vi "Draw_rounded_corners.vi"(7 "Corner scale  factor":dbl=0.1655 format="%#_13g", 8 "error in (no error)":errorcluster, 9 "Inner box coords":T1, 10 "Whole cage size, pix":cluster{"W":dbl, "H":dbl}, 11 "Refnum in":T2) -> (0 "error out":errorcluster, 3 "Refnum out":T2)   [LabVIEW 2018, in "Cage Diagram.lvlib"]
uses:
  Cage Diagram.lvlib
  <vilib>/vision/Image Controls.llb/IMAQ Image.ctl
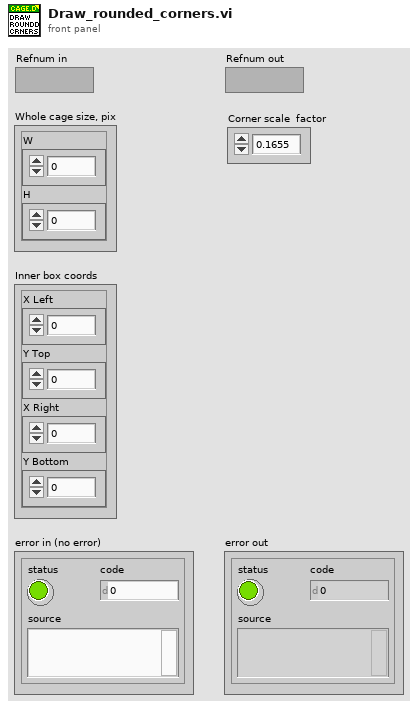
[diagram p1: front panel]
types:
  T1 = cluster{"X Left":dbl, "Y Top":dbl, "X Right":dbl, "Y Bottom":dbl}
  T2 = typedef "IMAQ Image.ctl" = refnum<image>
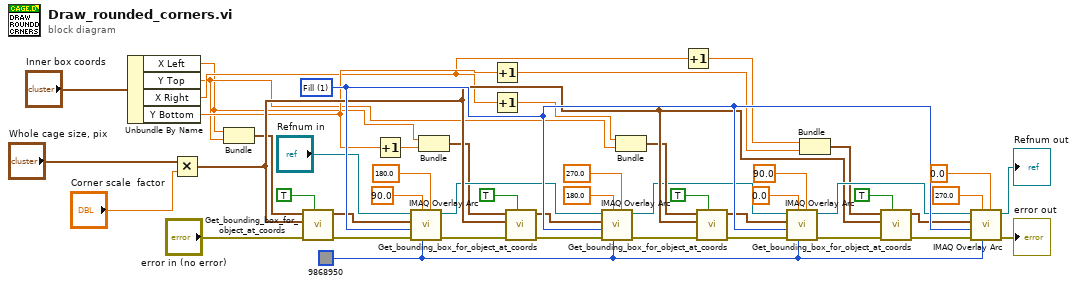
[diagram p0: block diagram]
diagram:
  w48 = u32 9868950 ("Color")
  w47 = u32 1 items=["Frame", "Fill"] ("Drawing Mode (Frame)")
  n1 = Unbundle By Name("Inner box coords") -> ("X Left"=w22:dbl, "Y Top"=w33:dbl, "X Right"=w41:dbl, "Y Bottom"=w42:dbl)
  n2 = Multiply(x="Whole cage size, pix", y="Corner scale  factor") -> (x*y=w43:cluster{"W":dbl, "H":dbl})
  n3 = Bundle("X Left"=w22, "Y Top"=w33) -> (w7:cluster{"X Left":dbl, "Y Top":dbl})  [unwired: 1 in]
  n4 = call "Get_bounding_box_for_object_at_coords.vi"("Treat size as Radius?"=TRUE, "Error In"="error in (no error)", "Object Size, pix"=w43, "Object Coords, pix"=w7) -> ("Error Out"=w9:errorcluster, "Object Bounding Box"=w13:T1)  [unwired: 6 in]
  n5 = Increment(x=w42) -> (x+1=w4:dbl)
  n6 = call "IMAQ Overlay Arc"("End Angle (degrees)"=180.0, "Color"=w48, "Start Angle (degrees)"=90.0, "error in (no error)"=w9, "Drawing Mode (Frame)"=w47, "Bounding Rectangle"=w13, "Image"="Refnum in") -> ("error out"=w24:errorcluster, "Image Out"=w23:T2)  [unwired: 3 in]
  n7 = Bundle("X Left"=w22, w4) -> (w21:cluster{"X Left":dbl, dbl})  [unwired: 1 in]
  n8 = Increment(x=w42) -> (x+1=w1:dbl)
  n9 = Increment(x=w41) -> (x+1=w3:dbl)
  n10 = call "Get_bounding_box_for_object_at_coords.vi"("Treat size as Radius?"=TRUE, "Error In"=w24, "Object Size, pix"=w43, "Object Coords, pix"=w21) -> ("Error Out"=w19:errorcluster, "Object Bounding Box"=w18:T1)  [unwired: 6 in]
  n11 = call "IMAQ Overlay Arc"("End Angle (degrees)"=270.0, "Color"=w48, "Start Angle (degrees)"=180.0, "error in (no error)"=w19, "Drawing Mode (Frame)"=w47, "Bounding Rectangle"=w18, "Image"=w23) -> ("error out"=w31:errorcluster, "Image Out"=w30:T2)  [unwired: 3 in]
  n12 = Bundle(w3, "Y Top"=w33) -> (w32:cluster{dbl, "Y Top":dbl})  [unwired: 1 in]
  n13 = Increment(x=w41) -> (x+1=w2:dbl)
  n14 = call "Get_bounding_box_for_object_at_coords.vi"("Treat size as Radius?"=TRUE, "Error In"=w31, "Object Size, pix"=w43, "Object Coords, pix"=w32) -> ("Error Out"=w26:errorcluster, "Object Bounding Box"=w27:T1)  [unwired: 6 in]
  n15 = call "IMAQ Overlay Arc"("End Angle (degrees)"=90.0, "Color"=w48, "Start Angle (degrees)"=0.0, "error in (no error)"=w26, "Drawing Mode (Frame)"=w47, "Bounding Rectangle"=w27, "Image"=w30) -> ("error out"=w45:errorcluster, "Image Out"=w44:T2)  [unwired: 3 in]
  n16 = Bundle(w2, w1) -> (w34:cluster{dbl, dbl})  [unwired: 1 in]
  n17 = call "Get_bounding_box_for_object_at_coords.vi"("Treat size as Radius?"=TRUE, "Error In"=w45, "Object Size, pix"=w43, "Object Coords, pix"=w34) -> ("Error Out"=w38:errorcluster, "Object Bounding Box"=w37:T1)  [unwired: 6 in]
  n18 = call "IMAQ Overlay Arc"("End Angle (degrees)"=0.0, "Color"=w48, "Start Angle (degrees)"=270.0, "error in (no error)"=w38, "Drawing Mode (Frame)"=w47, "Bounding Rectangle"=w37, "Image"=w44) -> ("error out"=→"error out":errorcluster, "Image Out"=→"Refnum out":T2)  [unwired: 3 in]
